vi "Add Controls in Configuration.vi"(0 "New Code Module":path, 1 "vi reference":refnum<vi>, 2 "Configuration Ctl Refnum":refnum<vi>, 11 "error in (no error)":errorcluster) -> (4 "Controls Reference":refnum<vi>[](array[refnum]), 15 "error out":errorcluster)   [LabVIEW 2021, in "Converter.lvlib"]
uses:
  Converter.lvlib
  Converter Reusables/Converter Reusables.lvlib
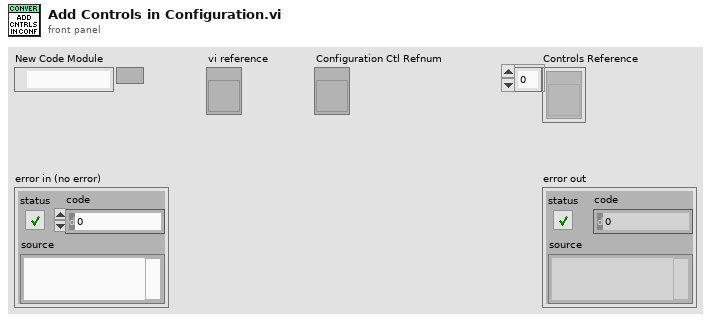
[diagram p1: front panel]
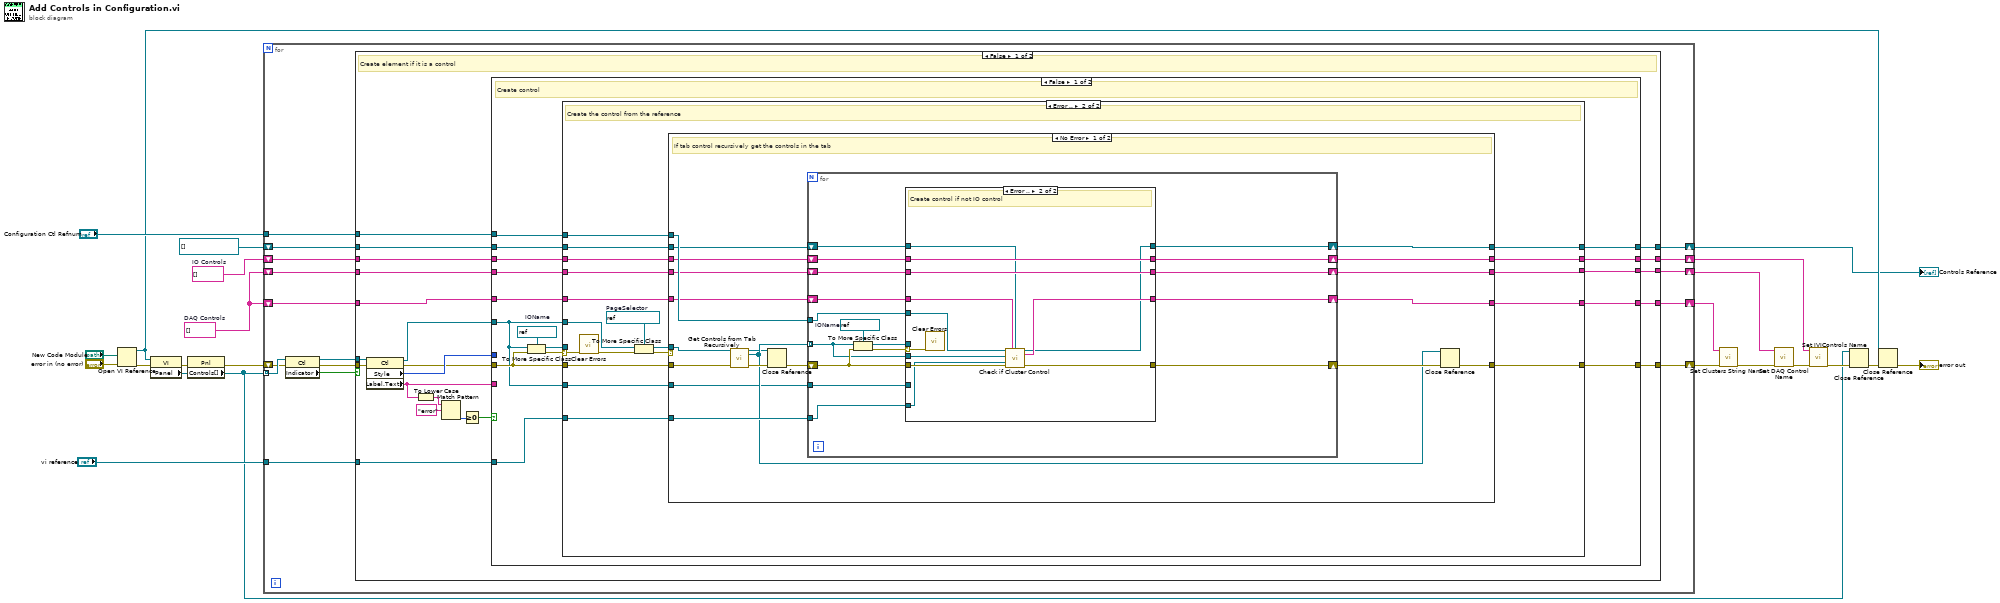
[diagram p0: block diagram]
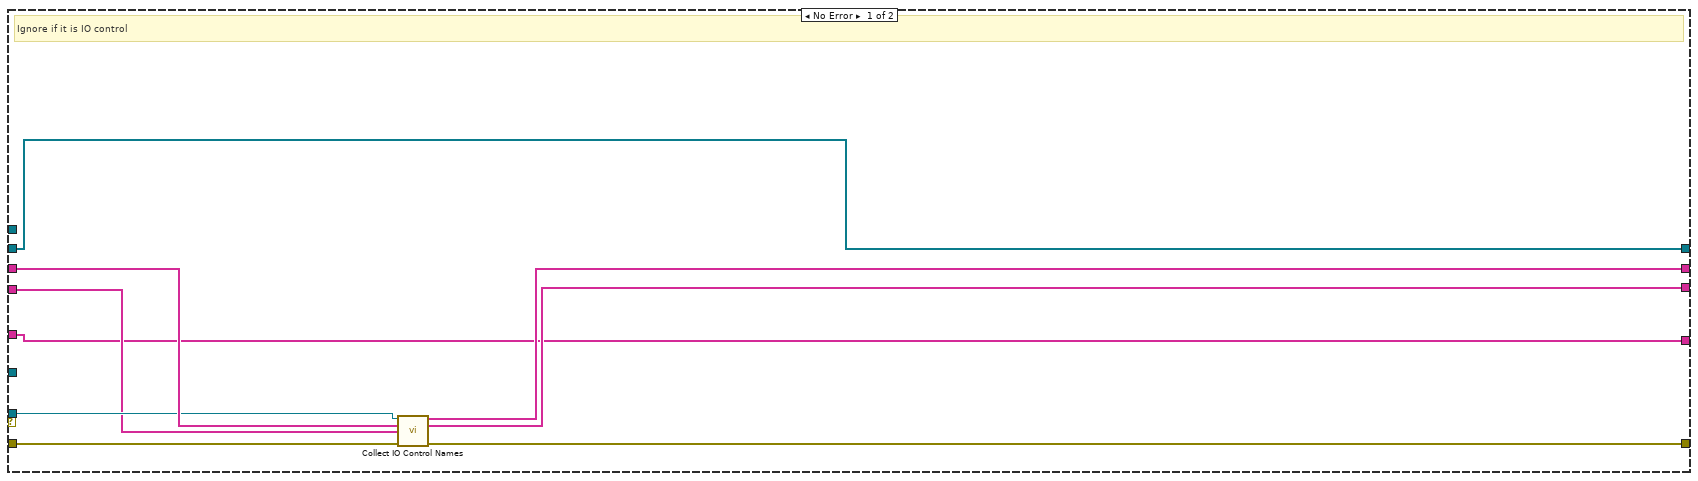
[diagram p2: hidden frame]
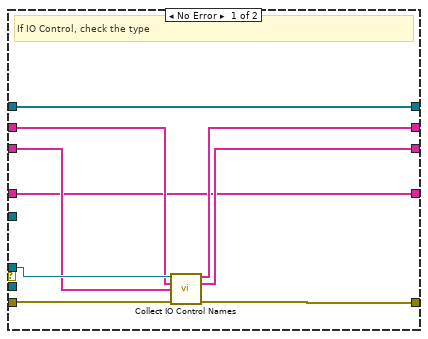
[diagram p3: hidden frame]
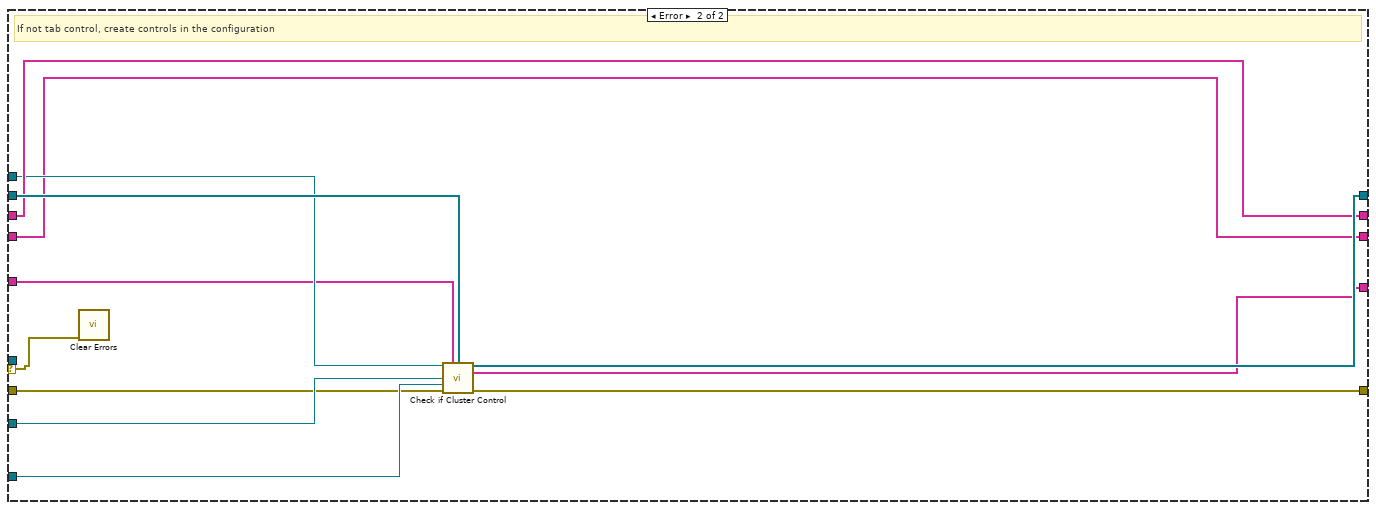
[diagram p4: hidden frame]
diagram:
  w4 = string[] []  # DAQ Controls
  w8 = string[] []  # IO Controls
  n1 = Open VI Reference(vi path="New Code Module", error in (no error)="error in (no error)") -> (vi reference=w14:refnum<vi>, error out=w12:errorcluster)  [unwired: 4 in]
  n2 = property class="VI"(reference=w14, error in=w12) -> (error out=w16:errorcluster, "Panel"=w15:refnum<vi>)  [unwired: 1 out]
  n3 = property class="Pnl"(reference=w15, error in=w16) -> (error out=w11:errorcluster, "Controls[]"=w13:refnum<vi>[])  [unwired: 1 out]
  n4 = for {
    tunnel: w13 -> [w37] mode=indexing
    shift-right: [w38] -> w1
    shift-left: w11 -> [w35]
    tunnel: "Configuration Ctl Refnum" -> [w39]
    tunnel: "vi reference" -> [w32]
    shift-right: [w31] -> w10
    shift-left: refnum<vi>[] [] -> [w30]
    shift-right: [w28] -> w9
    shift-left: w8 -> [w29]
    shift-right: [w26] -> w6
    shift-left: w4 -> [w27]
    shift-right: [w25] -> w3
    shift-left: w4 -> [w24]
    n5 = property class="Ctl"(reference=w37, error in=w35) -> (reference out=w33:refnum<vi>, error out=w34:errorcluster, "Indicator"=w36:bool)
    n6 = case shown="False" w36 {
      tunnel: w39 -> [w59 _]
      tunnel: w34 -> [w58 w183]
      tunnel: w33 -> [w56 _]
      tunnel: [w55 w183] -> w38
      tunnel: w32 -> [w48 _]
      tunnel: [w47 w182] -> w31
      tunnel: w30 -> [w46 w182]
      tunnel: w29 -> [w45 w181]
      tunnel: [w44 w181] -> w28
      tunnel: w27 -> [w43 w180]
      tunnel: [w42 w180] -> w26
      tunnel: [w41 w179] -> w25
      tunnel: w24 -> [w40 w179]
      frame False {
        # "Create element if it is a control"
        n7 = property class="Ctl"(reference=w56, error in=w58) -> (reference out=w49:refnum<vi>, error out=w57:errorcluster, "Style"=w60:u32, "Label.Text"=w54:string)
        n8 = To Lower Case(string=w54) -> (all lower case string=w50:string)
        n9 = Match Pattern(string=w50, regular expression="error") -> (offset past match=w52:i32)  [unwired: 1 in, 3 out]
        n10 = Greater Or Equal To 0?(x=w52) -> (x >= 0?=w51:bool)
        n11 = case shown="False" w51 {
          tunnel: w60 -> [_ _]
          tunnel: w59 -> [w74 _]
          tunnel: w57 -> [w76 w178]
          tunnel: w49 -> [w69 _]
          tunnel: w54 -> [_ _]
          tunnel: [w75 w178] -> w55
          tunnel: w48 -> [w73 _]
          tunnel: [w68 w177] -> w47
          tunnel: w46 -> [w67 w177]
          tunnel: w45 -> [w66 w176]
          tunnel: [w65 w176] -> w44
          tunnel: w43 -> [w64 w175]
          tunnel: [w63 w175] -> w42
          tunnel: [w62 w174] -> w41
          tunnel: w40 -> [w61 w174]
          frame False {
            w72 = refnum<vi> refnum  # IOName
            # "Create control"
            n12 = To More Specific Class(target class=w72, reference=w69, error in=w76) -> (specific class reference=w70:refnum<vi>, error out=w71:errorcluster)
            n13 = case shown="Error .." w71 {
              selector: w71 -> [_ w101]
              tunnel: w73 -> [_ w98]
              tunnel: w69 -> [_ w104]
              tunnel: w74 -> [_ w103]
              tunnel: [w85 w102] -> w75
              tunnel: w76 -> [w81 w100]
              tunnel: w70 -> [w80 _]
              tunnel: w69 -> [_ w96]
              tunnel: [w84 w93] -> w68
              tunnel: w67 -> [w84 w92]
              tunnel: w66 -> [w83 w91]
              tunnel: [w82 w90] -> w65
              tunnel: w64 -> [w79 w89]
              tunnel: [w78 w88] -> w63
              tunnel: [w77 w87] -> w62
              tunnel: w61 -> [w77 w86]
              frame No Error {
                # "Ignore if it is IO control"
                n14 = call "Collect IO Control Names.vi"("IO Control"=w80, "IO Controls in"=w83, "DAQ Controls in"=w79, "error in (no error)"=w81) -> ("IO Controls out"=w82:string[], "DAQ Controls out"=w78:string[], "error out"=w85:errorcluster)  [unwired: 9 in]
              }
              frame Error {
                w99 = refnum<vi> refnum  # PageSelector
                # "Create the control from the reference"
                n15 = call <vilib>:"Clear Errors.vi"("error in (no error)"=w101) -> ("error out"=w97:errorcluster)  [unwired: 5 in, 1 out]
                n16 = To More Specific Class(target class=w99, reference=w96, error in=w97) -> (specific class reference=w94:refnum<vi>, error out=w95:errorcluster)
                n17 = case shown="No Error" w95 {
                  selector: w95 -> [_ w163]
                  tunnel: w98 -> [w120 w170]
                  tunnel: w104 -> [w109 w167]
                  tunnel: w103 -> [w119 w168]
                  tunnel: [w123 w169] -> w102
                  tunnel: w100 -> [w122 w162]
                  tunnel: w94 -> [w121 _]
                  tunnel: [w107 w172] -> w93
                  tunnel: w92 -> [w108 w173]
                  tunnel: w91 -> [w118 w171]
                  tunnel: [w117 w171] -> w90
                  tunnel: w89 -> [w111 w166]
                  tunnel: [w110 w166] -> w88
                  tunnel: [w105 w165] -> w87
                  tunnel: w86 -> [w106 w164]
                  frame No Error {
                    # "If tab control recursively get the controls in the tab"
                    n18 = call "Get Controls from Tab Recursively.vi"("PageSel Refnum"=w121, "error in (no error)"=w122) -> ("Indicators in Tab"=w112:refnum<vi>[], "Controls in Tab"=w113:refnum<vi>[], "error out"=w115:errorcluster)  [unwired: 11 in]
                    n19 = Close Reference(reference=w112, error in (no error)=w115) -> (error out=w114:errorcluster)
                    n20 = for {
                      tunnel: w113 -> [w126] mode=indexing
                      tunnel: w120 -> [w129]
                      tunnel: w119 -> [w131]
                      shift-right: [w134] -> w117
                      shift-left: w118 -> [w138]
                      shift-right: [w135] -> w116
                      shift-left: w114 -> [w132]
                      shift-right: [w133] -> w110
                      shift-left: w111 -> [w136]
                      tunnel: w109 -> [w130]
                      shift-right: [w127] -> w107
                      shift-left: w108 -> [w128]
                      shift-right: [w124] -> w105
                      shift-left: w106 -> [w125]
                      w140 = refnum<vi> refnum  # IOName
                      n21 = To More Specific Class(target class=w140, reference=w126, error in=w132) -> (specific class reference=w139:refnum<vi>, error out=w137:errorcluster)
                      n22 = case shown="Error .." w137 {
                        selector: w137 -> [_ w159]
                        tunnel: w139 -> [w149 _]
                        tunnel: w138 -> [w148 w161]
                        tunnel: w136 -> [w147 w160]
                        tunnel: [w146 w154] -> w135
                        tunnel: [w145 w161] -> w134
                        tunnel: [w144 w160] -> w133
                        tunnel: w132 -> [w143 w155]
                        tunnel: w131 -> [_ w156]
                        tunnel: w130 -> [_ _]
                        tunnel: w129 -> [_ w152]
                        tunnel: [w142 w150] -> w127
                        tunnel: w128 -> [w142 w151]
                        tunnel: w126 -> [_ w153]
                        tunnel: w125 -> [w141 w158]
                        tunnel: [w141 w157] -> w124
                        frame No Error {
                          # "If IO Control, check the type"
                          n23 = call "Collect IO Control Names.vi"("IO Control"=w149, "IO Controls in"=w148, "DAQ Controls in"=w147, "error in (no error)"=w143) -> ("IO Controls out"=w145:string[], "DAQ Controls out"=w144:string[], "error out"=w146:errorcluster)  [unwired: 9 in]
                        }
                        frame Error {
                          # "Create control if not IO control"
                          n24 = call <vilib>:"Clear Errors.vi"("error in (no error)"=w159) -> ()  [unwired: 5 in, 2 out]
                          n25 = call "Check if Cluster Control.vi"("Typedef Cluster"=w156, "String Controls in"=w158, "Controls Ref IN"=w151, "Ctl Refnum"=w153, "vi reference"=w152, "error in"=w155) -> ("Controls Ref Out"=w150:refnum<vi>[], "String Controls out"=w157:string[], "error out"=w154:errorcluster)  [unwired: 7 in]
                        }
                      }
                    }
                    n26 = Close Reference(reference=w113, error in (no error)=w116) -> (error out=w123:errorcluster)
                  }
                  frame Error {
                    # "If not tab control, create controls in the configuration"
                    n27 = call <vilib>:"Clear Errors.vi"("error in (no error)"=w163) -> ()  [unwired: 5 in, 2 out]
                    n28 = call "Check if Cluster Control.vi"("Typedef Cluster"=w168, "String Controls in"=w164, "Controls Ref IN"=w173, "Ctl Refnum"=w167, "vi reference"=w170, "error in"=w162) -> ("Controls Ref Out"=w172:refnum<vi>[], "String Controls out"=w165:string[], "error out"=w169:errorcluster)  [unwired: 7 in]
                  }
                }
              }
            }
          }
          frame True {
            # "Ignore if it is error control"
          }
        }
      }
      frame True {
        # "Ignore if it is indicator"
      }
    }
  }
  "Controls Reference" <- w10
  n29 = call "Set Clusters String Name.vi"("Controls Name"=w3, "error in (no error)"=w1) -> ("error out"=w2:errorcluster)  [unwired: 13 in]
  n30 = call "Set DAQ Control Name.vi"("Controls Name"=w6, "error in (no error)"=w2) -> ("error out"=w5:errorcluster)  [unwired: 13 in]
  n31 = call "Set IVIControls Name.vi"("Controls Name"=w9, "error in (no error)"=w5) -> ("error out"=w18:errorcluster)  [unwired: 13 in]
  n32 = Close Reference(reference=w13, error in (no error)=w18) -> (error out=w20:errorcluster)
  n33 = Close Reference(reference=w14, error in (no error)=w20) -> (error out=→"error out":errorcluster)
